vi "HFRR ADV v025 new software.vi"() -> ()   [LabVIEW 2025] (continued)
              n2926 = Greater?(x=w4117, y=1) -> (0:w4113:bool)
            }
            n2927 = local write "String 29"(w4094) -> ()
            n2928 = Search and Replace String(input string=w4094, search string=".duf", replace string=".dgf" ("replace string (\"\")")) -> (result string=→"String Indicator 4":string)  [unwired: 5 in, 3 out]
            n2929 = Match Pattern(string=w4109, regular expression=".dwm") -> (before substring=w4093:string)  [unwired: 1 in, 3 out]
            "String Indicator" <- w4093
            n2930 = Match Pattern(string=w4094, regular expression=".dwm" ("substring (\"\")")) -> (before substring=w4095:string)  [unwired: 1 in, 3 out]
            "String Indicator 3" <- w4095
            n2931 = local write "TITTLE 2"(w4093) -> ()
            n2932 = String To Path(string=w4095) -> (path=w4102:path)
            "path" <- w4102
            n2933 = call <vilib>:"Read Characters From File.vi"("file path (dialog if empty)"=w4102, "start of read offset (chars.:0)"=60 ("start of read offset (chars.: 0)")) -> ("character string"=→"String Indicator 2":string)  [unwired: 4 in, 3 out]
          }
        }
        n2934 = call <vilib>:"Query Available Printers.vi"() -> ("system configured printers"=w3794:string[])  [unwired: 9 in, 2 out]
        "System Configured Printers 2" <- w3794
        n2935 = local read "OK Button 16"() -> (w3791:bool)
        n2936 = case shown="True" "OK Button 16" {
          frame False {
          }
          frame True {
            n2937 = stacked-sequence {
              frame #0 {
                n2938 = local read "Numeric 16"() -> (w4119:i32)
                n2939 = local write "Numeric 10"(w4119) -> ()
              }
              frame #1 {
                n2940 = local read "String 29"() -> (w4122:string)
                n2941 = String To Path(string=w4122) -> (path=w4121:path)
                n2942 = Open/Create/Replace File "Open File"(file path (use dialog)=w4121) -> (refnum out=w4123:refnum<file>)  [unwired: 5 in, 2 out]
                n2943 = for {
                  N: 16 -> [_]
                  tunnel: w4123 -> [w4130]
                  i -> [w4126]
                  (unwired) TRUE ("line mode (F)")
                  n2944 = Read from Text File "Read File"(file (use dialog)=w4130) -> (text=w4124:string)  [unwired: 3 in, 3 out]
                  n2945 = Match Pattern(string=w4124, regular expression="(") -> (after substring=w4129:string)  [unwired: 1 in, 3 out]
                  n2946 = Match Pattern(string=w4129, regular expression=")") -> (before substring=w4125:string)  [unwired: 1 in, 3 out]
                  n2947 = case shown="1" w4126 {
                    tunnel: w4125 -> [w4131 w4132 _ _ w4133 w4134 w4135 w4137 w4139 w4141 w4143 w4145 w4147 w4149 _]
                    tunnel: w4124 -> [_ _ _ _ _ _ _ _ _ _ _ _ _ _ _]
                    frame 0 {
                      "TITTLE" <- w4131
                    }
                    frame 1 {
                      "Sample ID" <- w4132
                    }
                    frame 2 {
                    }
                    frame 3 {
                    }
                    frame 4 {
                      "Test Date" <- w4133
                    }
                    frame 5 {
                      "Tested by" <- w4134
                    }
                    frame 6 {
                      n2948 = Fract/Exp String To Number(string=w4135) -> (number=→"Humidity before test 2":dbl)  [unwired: 3 in, 1 out]
                    }
                    frame 7 {
                      n2949 = Fract/Exp String To Number(string=w4137) -> (number=→"Temperature before test 2":dbl)  [unwired: 3 in, 1 out]
                    }
                    frame 8 {
                      n2950 = Fract/Exp String To Number(string=w4139) -> (number=→"Humidity after test 2":dbl)  [unwired: 3 in, 1 out]
                    }
                    frame 9 {
                      n2951 = Fract/Exp String To Number(string=w4141) -> (number=→"Temperature after test 2":dbl)  [unwired: 3 in, 1 out]
                    }
                    frame 10 {
                      n2952 = Fract/Exp String To Number(string=w4143) -> (number=→"MWSD 2":dbl)  [unwired: 3 in, 1 out]
                    }
                    frame 11 {
                      n2953 = Fract/Exp String To Number(string=w4145) -> (number=→"AVP 2":dbl)  [unwired: 3 in, 1 out]
                    }
                    frame 12 {
                      n2954 = Fract/Exp String To Number(string=w4147) -> (number=→"HCF 2":dbl)  [unwired: 3 in, 1 out]
                    }
                    frame 13 {
                      n2955 = Fract/Exp String To Number(string=w4149) -> (number=→"WS1.4 2":dbl)  [unwired: 3 in, 1 out]
                    }
                    frame 14, Default {
                    }
                  }
                }
              }
              frame #2 {
              }
            }
            n2956 = local write "OK Button 16"(FALSE ("OK Button 13")) -> ()
          }
        }
        n2957 = Index Array(array=w3794, index="Select Printer 3") -> (element=w3796:string)
        "Selected Printer" <- w3796
        n2958 = case shown="True" w3791 {
          frame False {
          }
          frame True {
            n2959 = flat-sequence {
              frame #0 {
              }
              frame #1 {
                n2960 = Wait (ms)(milliseconds to wait=u32 100) -> ()  [unwired: 1 out]
              }
              frame #2 {
                n2961 = local write "OK Button 16"(FALSE ("Print 3")) -> ()
              }
            }
          }
        }
        n2962 = case shown="True" "Print" {
          tunnel: w3796 -> [_ w4088]
          frame False {
          }
          frame True {
            (unwired) i16 6 ("width (-)")
            (unwired) "TESTED BY : "
            (unwired) "TESTED DATE :"
            (unwired) "SAMPLE ID : "
            (unwired) "SAMPLE DESIGN : "
            w4046 = "\r"
            w4063 = "\r"
            # "add image"
            n2963 = local read "Sample ID"() -> (w4036:string)
            n2964 = local read "Tested by"() -> (w4039:string)
            n2965 = local read "String 34"() -> (w4026:string)
            n2966 = local read "String 45"() -> (w4006:string)
            n2967 = local read "String 35"() -> (w4021:string)
            n2968 = local read "String 37"() -> (w4019:string)
            n2969 = local read "String 32"() -> (w4041:string)
            n2970 = local read "String 36"() -> (w4016:string)
            n2971 = local read "String 31"() -> (w4040:string)
            n2972 = local read "Test Date"() -> (w4037:string)
            n2973 = local read "String 33"() -> (w4042:string)
            n2974 = local read "String 38"() -> (w4012:string)
            n2975 = local read "String 39"() -> (w4009:string)
            n2976 = local write "Print"(FALSE ("Print FF")) -> ()
            n2977 = local read "S 39"() -> (w4024:string)
            n2978 = local read "S 38"() -> (w4031:string)
            n2979 = local read "Temperature before test 2"() -> (w4062:dbl)
            n2980 = local read "Temperature after test 2"() -> (w4052:dbl)
            n2981 = local read "Humidity before test 2"() -> (w4077:dbl)
            n2982 = local read "Humidity after test 2"() -> (w4061:dbl)
            n2983 = local read "MWSD 2"() -> (w4066:dbl)
            n2984 = local read "WS1.4 2"() -> (w4044:dbl)
            n2985 = Concatenate Strings("2)" ("string"), w4026) -> (w4027:string)
            n2986 = Concatenate Strings("3)" ("string"), w4024) -> (w4025:string)
            n2987 = Concatenate Strings("1)" ("string"), w4031) -> (w4030:string)
            n2988 = Concatenate Strings("4)" ("string"), w4021) -> (w4022:string)
            n2989 = Concatenate Strings("5)" ("string"), w4019) -> (w4018:string)
            n2990 = Concatenate Strings("6)" ("string"), w4016) -> (w4015:string)
            n2991 = Concatenate Strings("7)" ("string"), w4012) -> (w4013:string)
            n2992 = Concatenate Strings("8)" ("string"), w4009) -> (w4010:string)
            n2993 = local read "HCF 2"() -> (w4048:dbl)
            n2994 = local read "AVP 2"() -> (w4065:dbl)
            n2995 = local read "s.NO"() -> (w4007:string)
            n2996 = call <vilib>:"New Report.vi"("report type"=enum16{"Standard Report", "HTML"}."Standard Report") -> ("report out"=w4086:refnum<class "NI_report.lvclass">, "error out"=w4085:errorcluster)  [unwired: 13 in]
            n2997 = local read "TITTLE"() -> (w4038:string)
            n2998 = Concatenate Strings(w4063, w4006, w4007, w4063, w4041, w4036, w4063, w4040, w4037, w4063, w4042, w4039, w4063) -> (w4056:string)
            "test by" <- w4056
            n2999 = Number To Fractional String(number=w4062, width (-)=i16 6, precision (6)=i16 2) -> (F-format string=w4051:string)  [unwired: 1 in]
            n3000 = Number To Fractional String(number=w4061, width (-)=i16 6, precision (6)=i16 2) -> (F-format string=w4064:string)  [unwired: 1 in]
            n3001 = Number To Fractional String(number=w4077, width (-)=i16 6, precision (6)=i16 2) -> (F-format string=w4082:string)  [unwired: 1 in]
            n3002 = Number To Fractional String(number=w4066, width (-)=i16 6, precision (6)=i16 2) -> (F-format string=w4068:string)  [unwired: 1 in]
            n3003 = Number To Fractional String(number=w4052, width (-)=i16 6, precision (6)=i16 2) -> (F-format string=w4053:string)  [unwired: 1 in]
            n3004 = Number To Fractional String(number=w4065, width (-)=i16 6, precision (6)=i16 2) -> (F-format string=w4067:string)  [unwired: 1 in]
            n3005 = Number To Fractional String(number=w4048, width (-)=i16 6, precision (6)=i16 2) -> (F-format string=w4047:string)  [unwired: 1 in]
            n3006 = Number To Fractional String(number=w4044, precision (6)=i16 2) -> (F-format string=w4043:string)  [unwired: 2 in]
            n3007 = call-dynamic "Set Report Header Text.vi"("report in"=w4086, "center header text"=w4038, "error in (no error)"=w4085) -> ("report out"=w4057:refnum<class "NI_report.lvclass">, "error out"=w4058:errorcluster)  [unwired: 11 in]
            n3008 = Concatenate Strings(w4046, w4030, w4082, w4046, w4027, w4051, w4046, w4025, w4064, w4046, w4022, w4053, w4046, w4018, w4068, w4046, w4015, w4067, w4046, w4013, w4047, w4046, w4010, w4043) -> (w4034:string)
            "export 2" <- w4034
            n3009 = call-poly <vilib>:"Append Report Text.vi"("report in"=w4057, "text"=w4056, "error in (no error)"=w4058) -> ("report out"=w4060:refnum<class "NI_report.lvclass">, "error out"=w4059:errorcluster)  [unwired: 9 in, 2 out]
            n3010 = local read "test by"() -> (w4033:string)
            n3011 = local read "TITTLE"() -> (w4035:string)
            n3012 = call-poly <vilib>:"Append Report Text.vi"("report in"=w4060, "error in (no error)"=w4059) -> ("report out"=w4081:refnum<class "NI_report.lvclass">, "error out"=w4079:errorcluster)  [unwired: 10 in, 2 out]
            n3013 = Concatenate Strings(w4035, w4034, w4033) -> (→"output":string)
            n3014 = call-poly <vilib>:"Append Report Text.vi"("report in"=w4081, "text"=w4034, "error in (no error)"=w4079) -> ("report out"=w4080:refnum<class "NI_report.lvclass">, "error out"=w4078:errorcluster)  [unwired: 9 in, 2 out]
            n3015 = call-dynamic "Print Report.vi"("report in"=w4080, "printer name (default)"=w4088, "error in (no error)"=w4078) -> ("report out"=w4090:refnum<class "NI_report.lvclass">, "error out"=w4091:errorcluster)  [unwired: 11 in]
            n3016 = call-dynamic "Dispose Report.vi"("report in"=w4090, "error in (no error)"=w4091) -> ()  [unwired: 13 in, 1 out]
          }
        }
        n3017 = case shown="True" "Print 2" {
          frame False {
          }
          frame True {
            n3018 = flat-sequence {
              frame #0 {
                n3019 = local read "s.NO"() -> (→"s.NO 2":string)
                n3020 = Wait (ms)(milliseconds to wait=u32 20) -> ()  [unwired: 1 out]
                n3021 = local read "Sample ID  3"() -> (→"Sample ID  6":string)
                n3022 = local read "Sample ID  4"() -> (→"Sample ID  7":string)
                n3023 = local read "Sample ID"() -> (→"Sample ID  2":string)
                n3024 = local read "Tested by"() -> (→"Tested by 2":string)
                n3025 = local read "Test Date"() -> (→"Test Date 2":string)
                n3026 = local read "Humidity after test 3"() -> (→"Humidity after test 4":dbl)
                n3027 = local read "Ref A Test Date :"() -> (→"TITTLE 4":string)
                n3028 = local read "Temperature before test 3"() -> (w3913:dbl)
                n3029 = local read "Temperature before test 3"() -> (→"Temperature after test 5":dbl)
                n3030 = local read "Temperature after test 3"() -> (→"Temperature after test 4":dbl)
                n3031 = local read "Humidity before test 3"() -> (→"Humidity before test 4":dbl)
                n3032 = local write "Temperature before test 3"(w3913) -> ()
                n3033 = local read "image data"() -> (w3904:T14)
                n3034 = String To Path(string="C:\\LAB-IQ\\im\\Temp_resized.jpg") -> (path=w3905:path)
                "path 2" <- w3905
                n3035 = call <vilib>:"Write JPEG File.vi"("image data"=w3904, "path to JPEG file"=w3905) -> ()  [unwired: 8 in, 2 out]
                "Ref A Test Date :" <- "Ref A Test Date :"
                "Ref B Test Date :" <- "Ref B Test Date :"
                "Ref B Scar Value :" <- "Ref B Scar Value :"
                "Ref A Scar Value :" <- "Ref A Scar Value :"
              }
              frame #1 {
                (unwired) HTML_Report_Image_Alignment."MIDDLE" ("alignment (default)")
                w3941 = u16 0 items=["portrait", "landscape"] ("orientation (portrait)")
                (unwired) HTML_Report_Image_Alignment."ABSMIDDLE" ("alignment (default)")
                (unwired) "TESTED BY : "
                (unwired) "TESTED DATE :"
                (unwired) "SAMPLE ID : "
                (unwired) "SAMPLE DESIGN : "
                w3974 = "\r"
                # "add image"
                n3036 = Wait (ms)(milliseconds to wait=u32 20) -> ()  [unwired: 1 out]
                n3037 = local read "Sample ID  2"() -> (w3967:string)
                n3038 = local read "Wear Scar X"() -> (w3939:dbl)
                "Length ( microns ) 2" <- w3939
                n3039 = local read "Wear Scar Y"() -> (w3938:dbl)
                "Wear Scar Y ( microns ) :" <- w3938
                n3040 = local read "Test Date 2"() -> (w3968:string)
                n3041 = local read "Tested by 2"() -> (w3969:string)
                n3042 = local read "String 46"() -> (w3965:string)
                n3043 = local read "String 48"() -> (w3971:string)
                n3044 = local read "String 47"() -> (w3970:string)
                n3045 = local read "String 49"() -> (w3972:string)
                n3046 = local read "String 10"() -> (w3925:string)
                n3047 = local read "s.NO 2"() -> (w3966:string)
                n3048 = Add(x=w3939, y=w3938) -> (x+y=w3937:dbl)
                n3049 = call <vilib>:"New Report.vi"("report type"=enum16{"Standard Report", "HTML"}."HTML") -> ("report out"=w3945:refnum<class "NI_report.lvclass">, "error out"=w3943:errorcluster)  [unwired: 13 in]
                n3050 = Concatenate Strings(w3974, w3965, w3966, w3974, w3971, w3967, w3974, w3970, w3968, w3974, w3972, w3969, w3974) -> (→"test by 2":string)
                n3051 = Concatenate Strings("C:\\LAB-IQ\\Data\\" ("string"), w3925, ".jpg" ("string")) -> ()  [unwired: 1 out]
                n3052 = Divide(x=w3937, y=2.0) -> (x/y=→"Mean Wear ( microns) :":dbl)
                n3053 = call-dynamic "Set Report Orientation.vi"("report in"=w3945, "orientation (portrait)"=w3941, "error in (no error)"=w3943) -> ("report out"=w3944:refnum<class "NI_report.lvclass">, "error out"=w3942:errorcluster)  [unwired: 11 in]
                n3054 = for {
                  N: 5 -> [_]
                  tunnel: w3944 -> [w3995]
                  tunnel: [w3994] -> w3923
                  tunnel: w3942 -> [w3993]
                  tunnel: [w3992] -> w3922
                  n3055 = call-dynamic "Set Report Tab Width.vi"("report in"=w3995, "error in (no error)"=w3993) -> ("report out"=w3994:refnum<class "NI_report.lvclass">, "error out"=w3992:errorcluster)  [unwired: 12 in]
                }
                n3056 = local read "TITTLE"() -> (w3940:string)
                n3057 = call-dynamic "Set Report Header Text.vi"("report in"=w3923, "center header text"=w3940, "error in (no error)"=w3922) -> ("report out"=w3961:refnum<class "NI_report.lvclass">, "error out"=w3960:errorcluster)  [unwired: 11 in]
                n3058 = for {
                  N: 1 -> [_]
                  tunnel: [w3999] -> w3947
                  tunnel: [w3998] -> w3946
                  tunnel: w3961 -> [w3997]
                  tunnel: w3960 -> [w3996]
                  n3059 = call-dynamic "New Report Line.vi"("report in"=w3997, "error in (no error)"=w3996) -> ("report out"=w3999:refnum<class "NI_report.lvclass">, "error out"=w3998:errorcluster)  [unwired: 12 in]
                }
                n3060 = for {
                  N: 2 -> [_]
                  tunnel: [w3991] -> w3953
                  tunnel: [w3990] -> w3952
                  tunnel: w3947 -> [w3989]
                  tunnel: w3946 -> [w3988]
                  n3061 = call-dynamic "New Report Line.vi"("report in"=w3989, "error in (no error)"=w3988) -> ("report out"=w3991:refnum<class "NI_report.lvclass">, "error out"=w3990:errorcluster)  [unwired: 12 in]
                }
                n3062 = for {
                  N: 25 -> [_]
                  tunnel: w3953 -> [w3987]
                  tunnel: w3952 -> [w3985]
                  tunnel: [w3986] -> w3956
                  tunnel: [w3984] -> w3955
                  n3063 = call-dynamic "Set Report Tab Width.vi"("report in"=w3987, "error in (no error)"=w3985) -> ("report out"=w3986:refnum<class "NI_report.lvclass">, "error out"=w3984:errorcluster)  [unwired: 12 in]
                }
                n3064 = control-ref of="Tab Control 9"() -> (w3951:refnum<vi>)
                n3065 = call-dynamic "Append Control Image to Report.vi"("report in"=w3956, "alignment (default)"=HTML_Report_Image_Alignment."ABSMIDDLE", "ctrl reference"=w3951, "error in (no error)"=w3955) -> ("report out"=w3950:refnum<class "NI_report.lvclass">, "error out"=w3949:errorcluster)  [unwired: 8 in, 2 out]
                n3066 = for {
                  N: 3 -> [_]
                  tunnel: [w3983] -> w3934
                  tunnel: [w3982] -> w3933
                  tunnel: w3950 -> [w3981]
                  tunnel: w3949 -> [w3980]
                  n3067 = call-dynamic "New Report Line.vi"("report in"=w3981, "error in (no error)"=w3980) -> ("report out"=w3983:refnum<class "NI_report.lvclass">, "error out"=w3982:errorcluster)  [unwired: 12 in]
                }
                n3068 = for {
                  N: 100 -> [_]
                  tunnel: w3934 -> [w3979]
                  tunnel: w3933 -> [w3977]
                  tunnel: [w3978] -> w3930
                  tunnel: [w3976] -> w3928
                  n3069 = call-dynamic "Set Report Tab Width.vi"("report in"=w3979, "error in (no error)"=w3977) -> ("report out"=w3978:refnum<class "NI_report.lvclass">, "error out"=w3976:errorcluster)  [unwired: 12 in]
                }
                n3070 = String To Path(string="C:\\LAB-IQ\\im\\Temp_resized.jpg") -> (path=w3920:path)
                n3071 = call-poly <vilib>:"Append Image to Report.vi"("report in"=w3930, "path or URL of image"=w3920, "error in (no error)"=w3928) -> ("report out"=w3929:refnum<class "NI_report.lvclass">, "error out"=w3927:errorcluster)  [unwired: 9 in, 2 out]
                n3072 = call-poly <vilib>:"Open HTML Report in Browser.vi"("report in"=w3929, "error in (no error)"=w3927) -> ("report out"=w3964:refnum<class "NI_report.lvclass">, "error out"=w3963:errorcluster)  [unwired: 11 in, 1 out]
                n3073 = call-dynamic "Dispose Report.vi"("report in"=w3964, "error in (no error)"=w3963) -> ()  [unwired: 13 in, 1 out]
              }
              frame #2 {
              }
              frame #3 {
                n3074 = disable-structure shown="Disabled" {
                  frame Disabled {
                    n3075 = local read "String 10"() -> (w4004:string)
                    n3076 = Concatenate Strings("C:\\LAB-IQ-NXT\\Data\\" ("string"), w4004, ".jpg" ("string")) -> (w4002:string)
                    n3077 = String To Path(string=w4002) -> (path=w4001:path)
                    n3078 = Delete(path (use dialog)=w4001) -> ()  [unwired: 4 in, 3 out]
                  }
                  frame Enabled {
                  }
                }
                n3079 = local write "Print 2"(FALSE ("Print")) -> ()
              }
            }
          }
        }
      }
    }
    n3080 = property on="SetTemp" class="DigNum (strict)"("Disabled"=w2100) -> ()  [unwired: 2 in, 2 out]
    n3081 = Multiply(x=w2090, y=w2092) -> (x*y=w2091:dbl)
    n3082 = local read "MWSD"() -> (w2089:dbl)
    n3083 = Add(x=w2091, y=w2089) -> (x+y=→"WS1.4":dbl)
    n3084 = Wait (ms)(milliseconds to wait=u32 50) -> ()  [unwired: 1 out]
    n3085 = Wait (ms)(milliseconds to wait=u32 50) -> ()  [unwired: 1 out]
    n3086 = local read "Quit"() -> (w2088:bool)
  }
  n3087 = VISA Close(VISA resource name=w41, error in (no error)=w40) -> ()  [unwired: 1 out]
  n3088 = while {
    tunnel: [w4164] -> w50
    shift-right: [w4157] -> _
    shift-left: 0.0 -> [w4160]
    shift-right: [w4156] -> _
    shift-left: 0.0 -> [w4159]
    shift-right: [w4155] -> _
    shift-left: 100.0 ("vc_cmd") -> [w4158]
    stop <- w4164 stop-if-true
    # "PID LOGIC"
    n3089 = local read "RUN"() -> (w4162:bool)
    n3090 = local read "Auto Start Temp"() -> (w4151:bool)
    n3091 = local read "Auto Start Test"() -> (w4161:bool)
    n3092 = local read "START TEMP"() -> (w4153:bool)
    n3093 = And(x=w4151, y=w4161) -> (x .and. y?=w4152:bool)
    n3094 = Or(x=w4162, y=w4152) -> (x .or. y?=w4163:bool)
    n3095 = And(x=w4163, y=w4153) -> (x .and. y?=w4154:bool)
    n3096 = Wait (ms)(milliseconds to wait="milliseconds to wait") -> ()  [unwired: 1 out]
    n3097 = case shown="True" w4154 {
      tunnel: [400.0 ("out_vc_cmd") w4184] -> w4155
      tunnel: [w4167 w4186] -> w4156
      tunnel: [w4167 w4185] -> w4157
      tunnel: w4160 -> [_ w4175]
      tunnel: w4159 -> [_ w4174]
      tunnel: w4158 -> [_ w4173]
      frame False {
        w4167 = 0.0 ("error_out")
      }
      frame True {
        n3098 = local read "Set Strk"() -> (w4170:dbl)
        n3099 = local read "LVDT STROKE"() -> (w4168:dbl)
        n3100 = Add(x=w4170, y="Add up Stroke") -> (x+y=w4171:dbl)
        n3101 = formula code="// Zero-Hardcode Explicit Positional-Form PID Engine\n// Inputs: target_stroke, measured_stroke, dt, prev_error, integral_accumulator_in, prev_vc_cmd\n//         kp, ki, kd, max_step_change, max_amplitude, min_amplitude, startup_cmd\n// Outputs: vc_cmd, error_out, out_error, integral_accumulator_out, out_vc_cmd\n\n// 1. Calculate Tracking Error\nfloat current_error = target_stroke - measured_stroke;\nerror_out = current_error;\n\n// 2. Compute Proportional Term\nfloat p_term = kp * current_error;\n\n// 3. Compute Derivative Term\nfloat d_term = 0.0;\nif (dt > 0.0) {\n    d_term = kd * ((current_error - prev_error) / dt);\n}\n\n// 4. Update and Accumulate Integral Term\nfloat current_integral = integral_accumulator_in + (current_error * dt);\nfloat i_term = ki * current_integral;\n\n// 5. Calculate Ideal Target Command\nfloat ideal_command = startup_cmd + p_term + i_term + d_term;\n\n// 6. Anti-Windup Protection (Back-calculation method)\nif (ideal_command > max_amplitude) {\n    float excess = ideal_command - max_amplitude;\n    if (ki > 0.0) {\n        current_integral -= excess / ki;\n    }\n    ideal_command = max_amplitude;\n} else if (ideal_command < min_amplitude) {\n    float excess = ideal_command - min_amplitude;\n    if (ki > 0.0) {\n        current_integral -= excess / ki;\n    }\n    ideal_command = min_amplitude;\n}\n\n// 7. Apply Loop Rate Limiting (Protects voice coil from large voltage steps)\nfloat raw_adjustment = ideal_command - prev_vc_cmd;\n\nif (raw_adjustment > max_step_change) {\n    raw_adjustment = max_step_change;\n} else if (raw_adjustment < -max_step_change) {\n    raw_adjustment = -max_step_change;\n}\n\nfloat next_vc_cmd = prev_vc_cmd + raw_adjustment;\n\n// Final Output Safety Safeguard Clamping\nif (next_vc_cmd > max_amplitude) {\n    next_vc_cmd = max_amplitude;\n} else if (next_vc_cmd < min_amplitude) {\n    next_vc_cmd = min_amplitude;\n}\n\n// 8. Map to Shift Registers for memory persistence\nvc_cmd = next_vc_cmd;\nout_error = current_error;                     \nintegral_accumulator_out = current_integral;  \nout_vc_cmd = next_vc_cmd;"("target_stroke"=w4171, "measured_stroke"=w4168, "dt"="dt", "integral_accumulator_in"=w4174, "prev_error"=w4175, "prev_vc_cmd"=w4173, "kp"="kp", "ki"="ki", "kd"="kd", "max_step_change"="max_step_change", "max_amplitude"="max_amplitude", "min_amplitude"="min_amplitude", "startup_cmd"="startup_cmd") -> ("vc_cmd"=w4190:dbl, "out_error"=w4185:dbl, "integral_accumulator_out"=w4186:dbl, "out_vc_cmd"=w4184:dbl)  [unwired: 1 out]
        "output Vpp" <- w4190
        n3102 = Number To Fractional String(number=w4190, precision (6)=i16 1) -> (F-format string=w4188:string)  [unwired: 2 in]
        n3103 = Concatenate Strings("DAC;" ("string"), w4188) -> (w4172:string)
        n3104 = local write "Due Write"(w4172) -> ()
        "prev_error" <- w4175
        "integral_accumulator_in" <- w4174
        "prev_vc_cmd" <- w4173
      }
    }
    n3105 = local read "Quit"() -> (w4164:bool)
  }
  n3106 = Or(x=w46, y=w45) -> (x .or. y?=w47:bool)
  n3107 = Or(x=w43, y=w47) -> (x .or. y?=w52:bool)
  n3108 = control-ref of="new picture"() -> ()  [unwired: 1 out]
  n3109 = Or(x=w55, y=w52) -> (x .or. y?=w49:bool)
  n3110 = Or(x=w49, y=w50) -> (x .or. y?=w44:bool)
  n3111 = while {
    tunnel: [w4191] -> w54
    i -> [w4198]
    stop <- w4191 stop-if-true
    n3112 = local read "Quit"() -> (w4191:bool)
    n3113 = Equal To 0?(x=w4198) -> (x = 0?=w4196:bool)
    n3114 = call "Elapsed Time3"("Time Target (s)"=45.0, "Auto Reset"=TRUE) -> ("Time has Elapsed"=w4195:bool)  [unwired: 10 in, 7 out]
    n3115 = Wait (ms)(milliseconds to wait=u32 50) -> ()  [unwired: 1 out]
    n3116 = Or(x=w4195, y=w4196) -> (x .or. y?=w4197:bool)
    n3117 = case shown="True" w4197 {
      frame False {
      }
      frame True {
        n3118 = call <vilib>:"System Exec.vi"("run minimized? (F)"=TRUE, "error in (no error)"="error in (no error)", "command line"="powercfg.exe -change -monitor-timeout-ac 0") -> ("error out"=w4209:errorcluster)  [unwired: 5 in, 3 out]
        n3119 = call <vilib>:"System Exec.vi"("run minimized? (F)"=TRUE, "error in (no error)"=w4209, "command line"="powercfg.exe -change -disk-timeout-ac 0") -> ("error out"=w4208:errorcluster)  [unwired: 5 in, 3 out]
        n3120 = call <vilib>:"System Exec.vi"("run minimized? (F)"=TRUE, "error in (no error)"=w4208, "command line"="powercfg.exe -change -standby-timeout-ac 0") -> ("error out"=w4207:errorcluster)  [unwired: 5 in, 3 out]
        n3121 = call <vilib>:"System Exec.vi"("run minimized? (F)"=TRUE, "error in (no error)"=w4207, "command line"="powercfg.exe -change -hibernate-timeout-ac 0") -> ("error out"=w4206:errorcluster)  [unwired: 5 in, 3 out]
        n3122 = call <vilib>:"Simple Error Handler.vi"("error in (no error)"=w4206) -> ("error out"=w4212:errorcluster)  [unwired: 4 in, 4 out]
        n3123 = call <vilib>:"Clear Errors.vi"("error in (no error)"=w4212) -> ("error out"=→"error out":errorcluster)  [unwired: 5 in, 1 out]
      }
    }
  }
  n3124 = Compound Arithmetic op=OR(w57, w44, w54) -> (w56:bool)
  n3125 = flat-sequence {
    tunnel: w56 -> [_]
    tunnel: [w4214] -> w25
    tunnel: w25 -> [_]
    frame #0 {
      n3126 = call "CLOSE CONNECTION.vi"() -> ("error out"=w4214:errorcluster)  [unwired: 11 in]
    }
    frame #1 {
      n3127 = Quit LabVIEW(quit? (T)=TRUE) -> ()
      n3128 = local write "Quit"(FALSE ("EXIT")) -> ()
    }
  }
  n3129 = property on="Heater Button" class="Bool (strict)"("Visible"=TRUE) -> ()  [unwired: 2 in, 2 out]
  n3130 = disable-structure shown="Disabled" {
    disable-tunnel: _ -> [w4220 _]
    disable-tunnel: _ -> [w4217 _]
    disable-tunnel: _ -> [w4218 _]
    frame Disabled {
      n3131 = disable-structure shown="Disabled" {
        disable-tunnel: [w4227 _] -> w4219
        frame Disabled {
          n3132 = while {
            shift-right: [w4269] -> w4225
            shift-left: errorcluster {"status"=TRUE, "code"=0, "source"="Init"} ("error out") -> [w4234]
            shift-right: [w4268] -> w4224
            shift-left: _ -> [w4235]
            shift-right: [w4267] -> _
            shift-left: "" -> [w4266]
            tunnel: [w4228] -> w4227
            shift-right: ["Set Rh"] -> _
            shift-left: 0.0 ("Set Rh") -> [w4260]
            tunnel: [w4237] -> _
            i -> [w4237]
            stop <- w4228 stop-if-true
            n3133 = flat-sequence {
              tunnel: w4234 -> [w4272]
              tunnel: [w4272] -> w4233
              frame #0 {
                n3134 = Wait (ms)(milliseconds to wait=u32 200) -> ()  [unwired: 1 out]
              }
            }
            n3135 = local read "Com Port 3"() -> (w4236:refnum<visa-resource-name>)
            n3136 = local read "Humidity Str Rec"() -> (w4238:string)
            n3137 = Not Equal?(x="Set Rh", y=w4260) -> (x != y?=w4265:bool)
            n3138 = Number To Decimal String(number="Set Rh") -> (decimal integer string=w4263:string)  [unwired: 1 in]
            n3139 = Not Equal?(x=w4236, y=w4235) -> (x != y?=w4231:bool)
            n3140 = Concatenate Strings("#setPoint00" ("string"), w4263) -> (w4264:string)
            n3141 = case shown="False" w4265 {
              tunnel: w4264 -> [_ w4284]
              frame False {
                n3142 = local read "Humidity"() -> (w4281:bool)
                n3143 = case shown="True" w4281 {
                  frame False {
                    n3144 = local write "Humidity Str Send"("stop" ("Humidity Str Send")) -> ()
                  }
                  frame True {
                    n3145 = local write "Humidity Str Send"("start" ("Humidity Str Send")) -> ()
                  }
                }
              }
              frame True {
                n3146 = local write "Humidity Str Send"(w4284) -> ()
              }
            }
            n3147 = Or(x=w4231) -> (y=w4229:bool, x .or. y?=w4230:bool)
            n3148 = String Subset(string=w4238, offset (0)=7) -> (substring=w4253:string)  [unwired: 1 in]
            n3149 = Match Pattern(string=w4238, regular expression="?") -> (offset past match=w4256:i32)  [unwired: 1 in, 3 out]
            n3150 = Match Pattern(string=w4238, regular expression="v") -> (offset past match=w4259:i32)  [unwired: 1 in, 3 out]
            n3151 = case shown="True" w4230 {
              tunnel: w4233 -> [w4270 _]
              tunnel: [w4270 errorcluster {"status"=TRUE, "code"=0, "source"="Init"} ("error out")] -> w4232
              frame False {
              }
              frame True {
              }
            }
            n3152 = Equal?(x=w4256, y=-1) -> (x = y?=w4240:bool)
            n3153 = Match Pattern(string=w4253, regular expression="g") -> (after substring=w4254:string, offset past match=w4245:i32)  [unwired: 1 in, 2 out]
            n3154 = Match Pattern(string=w4253, regular expression="y") -> (after substring=w4252:string, offset past match=w4246:i32)  [unwired: 1 in, 2 out]
            n3155 = Greater?(x=w4246, y=w4245) -> (0:w4251:bool)
            n3156 = Greater Or Equal To 0?(x=w4246) -> (x >= 0?=w4243:bool)
            n3157 = Greater Or Equal To 0?(x=w4245) -> (x >= 0?=w4244:bool)
            n3158 = Or(x=w4243, y=w4244) -> (x .or. y?=w4242:bool)
            n3159 = Greater Or Equal To 0?(x=w4259) -> (x >= 0?=w4241:bool)
            n3160 = Select(t=w4252, s=w4251, f=w4254) -> (s? t:f=w4247:string)
            n3161 = case shown="Error" w4232 {
              selector: w4232 -> [w4297 w4343]
              tunnel: [w4295 w4336] -> w4269
              tunnel: w4235 -> [w4298 w4342]
              tunnel: [w4296 w4345] -> w4268
              tunnel: w4266 -> [w4285 w4344]
              tunnel: [w4292 w4344] -> w4267
              frame No Error {
                n3162 = call "Elapsed Time7"() -> ("Time has Elapsed"=w4291:bool)  [unwired: 12 in, 7 out]
                n3163 = Not Equal?(x="Humidity Str Send", y=w4285) -> (x != y?=w4287:bool)
                n3164 = Or(x=w4287, y=w4291) -> (x .or. y?=w4290:bool)
                n3165 = Select(t="Humidity Str Send", s=w4287, f="vals" ("regular expression")) -> (s? t:f=w4286:string)
                n3166 = Or(x=w4290, y="Send") -> (x .or. y?=w4294:bool)
                n3167 = case shown="True" w4294 {
                  tunnel: [w4301 w4306] -> w4295
                  tunnel: w4298 -> [w4300 w4314]
                  tunnel: w4297 -> [w4301 w4313]
                  tunnel: [w4300 w4307] -> w4296
                  tunnel: w4286 -> [_ w4312]
                  tunnel: [w4299 w4303] -> w4292
                  tunnel: "Humidity Str Send" -> [_ w4304]
                  tunnel: w4287 -> [_ w4305]
                  tunnel: w4285 -> [w4299 w4302]
                  frame False {
                  }
                  frame True {
                    n3168 = flat-sequence {
                      tunnel: w4314 -> [w4322]
                      tunnel: w4313 -> [w4321]
                      tunnel: w4312 -> [w4318]
                      tunnel: [w4320] -> w4311
                      tunnel: [w4319] -> w4310
                      tunnel: w4311 -> [w4325]
                      tunnel: w4310 -> [w4324]
                      tunnel: [w4325] -> w4309
                      tunnel: [w4324] -> w4308
                      tunnel: w4309 -> [w4332]
                      tunnel: w4308 -> [w4331]
                      tunnel: [w4330] -> w4307
                      tunnel: [w4329] -> w4306
                      frame #0 {
                        n3169 = local write "Ser Led"(TRUE ("Boolean 4")) -> ()
                        n3170 = Concatenate Strings(w4318, "\r") -> (w4317:string)
                        n3171 = VISA Write(VISA resource name=w4322, write buffer=w4317, error in (no error)=w4321) -> (VISA resource name out=w4320:refnum<visa-resource-name>, error out=w4319:errorcluster)  [unwired: 1 out]
                      }
                      frame #1 {
                        n3172 = Wait (ms)(milliseconds to wait="wait") -> ()  [unwired: 1 out]
                      }
                      frame #2 {
                        w4327 = FALSE ("Send")
                        n3173 = property class="Instr"(reference=w4332, error in=w4331) -> (reference out=w4333:refnum<visa-resource-name>, error out=w4334:errorcluster, "Serial Settings:Number of Bytes at Serial Port"=w4326:u32)
                        n3174 = local write "Send"(w4327) -> ()
                        n3175 = local write "Ser Led"(w4327) -> ()
                        n3176 = VISA Read(VISA resource name=w4333, byte count=w4326, error in (no error)=w4334) -> (VISA resource name out=w4330:refnum<visa-resource-name>, read buffer=→"Humidity Str Rec":string, error out=w4329:errorcluster)  [unwired: 1 out]
                      }
                    }
                    n3177 = Select(t=w4304, s=w4305, f=w4302) -> (s? t:f=w4303:string)
                  }
                }
              }
              frame Error {
                w4350 = u16 0 items=["None"=0, "XON/XOFF"=1, "RTS/CTS"=2, "DTR/DSR"=4] ("flow control")
                w4346 = u16 0 items=["None", "Odd", "Even", "Mark", "Space"] ("parity")
                w4349 = u16 10 items=["1.0"=10, "1.5"=15, "2.0"=20] ("stop bits")
                n3178 = VISA Close(VISA resource name=w4342, error in (no error)=w4343) -> (error out=w4341:errorcluster)
                n3179 = local write "humid"("" ("humid")) -> ()
                n3180 = local write "Humidity Str Rec"("" ("Humidity Str Rec")) -> ()
                n3181 = call <vilib>:"Clear Errors.vi"("error in (no error)"=w4341) -> ("error out"=w4340:errorcluster)  [unwired: 5 in, 1 out]
                n3182 = local read "Com Port 3"() -> (w4339:refnum<visa-resource-name>)
                n3183 = call-poly "VISA Configure Serial Port"("VISA resource name"=w4339, "timeout (10sec)"=u32 1000, "termination char\n(0xA = '\\n' = LF)"=u8 10 ("termination char\n(0xA = '\\n' = LF)"), "Enable Termination\nChar (T)"=FALSE ("Enable Termination Char (T)"), "data bits (8)"=u16 8 ("data bits"), "parity (0:none)"=w4346, "error in (no error)"=w4340, "stop bits (10: 1 bit)"=w4349, "flow control (0:none)"=w4350) -> ("VISA resource name out"=w4345:refnum<visa-resource-name>, "baud rate (9600)"=w4337:u32, "error out"=w4336:errorcluster)  [unwired: 4 in]
              }
            }
            n3184 = Compound Arithmetic op=AND(w4241, w4240, w4242) -> (w4239:bool)
            n3185 = case shown="True" w4239 {
              tunnel: w4238 -> [_ _]
              tunnel: w4247 -> [_ w4277]
              frame False {
              }
              frame True {
                w4275 = " " ("regular expression")
                n3186 = Match Pattern(string=w4277, regular expression=" ") -> (after substring=w4279:string)  [unwired: 1 in, 3 out]
                n3187 = Match Pattern(string=w4279, regular expression=w4275) -> (before substring=→"humid":string, after substring=w4276:string)  [unwired: 1 in, 2 out]
                n3188 = Match Pattern(string=w4276, regular expression=w4275) -> (before substring=→"temp_@Rh sensor":string)  [unwired: 1 in, 3 out]
              }
            }
            n3189 = local read "Quit"() -> (w4228:bool)
          }
          n3190 = VISA Close(VISA resource name=w4224, error in (no error)=w4225) -> (error out=w4221:errorcluster)
          n3191 = call <vilib>:"Clear Errors.vi"("error in (no error)"=w4221) -> ()  [unwired: 5 in, 2 out]
        }
        frame Enabled {
        }
      }
    }
    frame Enabled {
    }
  }
  n3192 = while {
    tunnel: [w4357] -> _
    i -> [w4357]
    stop <- w4353 stop-if-true
    # "Langauage selection"
    n3193 = Equal?(x="Lan flag", y=22.0) -> ()  [unwired: 1 out]
    n3194 = disable-structure shown="Disabled" {
      frame Disabled {
        n3195 = stacked-sequence {
          frame #0 {
            n3196 = case shown="\"Russian\"" "Language Selection" {
              tunnel: [0 1] -> w4359
              frame "English", Default {
              }
              frame "Russian" {
              }
            }
            n3197 = for {
              N: 130 -> [_]
              tunnel: "Table" -> [w4368]
              tunnel: w4359 -> [w4367]
              i -> [w4366]
              n3198 = Index Array(array=w4368, index (row)=w4366, index (col)=w4367) -> (element=w4365:string)
              n3199 = case shown="123" w4366 {
                tunnel: w4365 -> [w4369 w4370 _ w4371 w4372 w4373 w4374 w4375 w4376 w4377 w4378 w4379 w4380 w4381 w4382 w4383 w4384 w4385 w4386 w4387 w4388 w4389 w4390 w4391 w4392 w4393 w4394 w4395 w4396 _ _ w4397 w4398 w4399 w4400 w4401 w4402 w4411 w4418 w4425 w4432 w4436 w4439 w4442 w4444 w4446 w4447 w4448 w4449 w4450 w4451 w4452 w4453 w4454 w4455 w4456 w4457 w4458 w4459 w4460 w4461 w4462 w4463 w4464 w4465 w4466 w4467 w4468 w4469 w4470 w4471 w4472 w4473 w4474 w4475 w4476 w4477 w4478 w4479 w4480 w4481 w4482 w4483 w4484 w4485 w4486 w4487 w4488 w4489 w4490 w4491 w4492 w4493 w4494 w4495 w4496 w4497 w4498 w4499 w4500 w4501 w4502 w4503 w4504 w4505 _ w4506 w4507 w4508 w4509 w4510 w4511 w4512 w4513 w4514 w4515 w4516 w4517 w4518 _ w4519 w4520 w4521 w4522 w4523 w4524 _]
                frame 0 {
                  n3200 = local write "S"(w4369) -> ()
                }
                frame 1 {
                  n3201 = local write "S 2"(w4370) -> ()
                }
                frame 2 {
                }
                frame 3 {
                  n3202 = local write "S 4"(w4371) -> ()
                }
                frame 4 {
                  n3203 = property on="FILE" class="Str"("Caption.Text"=w4372) -> ()  [unwired: 2 in, 2 out]
                }
                frame 5 {
                  n3204 = property on="Fuel Discription :" class="Str"("Caption.Text"=w4373) -> ()  [unwired: 2 in, 2 out]
                }
                frame 6 {
                  n3205 = property on="Remarks :" class="Str"("Caption.Text"=w4374) -> ()  [unwired: 2 in, 2 out]
                }
                frame 7 {
                  n3206 = property on="Save & Continue" class="Bool (strict)"("Boolean Text.Text"=w4375) -> ()  [unwired: 2 in, 2 out]
                }
                frame 8 {
                }
                frame 9 {
                  n3207 = property on="Set Hz" class="DigNum (strict)"("Caption.Text"=w4377) -> ()  [unwired: 2 in, 2 out]
                }
                frame 10 {
                }
                frame 11 {
                  n3208 = property on="NORMAL LOAD" class="DigNum (strict)"("Caption.Text"=w4379) -> ()  [unwired: 2 in, 2 out]
                }
                frame 12 {
                }
                frame 13 {
                  n3209 = property on="Set Temp" class="DigNum (strict)"("Caption.Text"=w4381) -> ()  [unwired: 2 in, 2 out]
                }
                frame 14 {
                  n3210 = local write "S 15"(w4382) -> ()
                }
                frame 15 {
                  n3211 = property on="Set Rh" class="DigNum (strict)"("Caption.Text"=w4383) -> ()  [unwired: 2 in, 2 out]
                }
                frame 16 {
                }
                frame 17 {
                  n3212 = local write "S 18"(w4385) -> ()
                }
                frame 18 {
                  "String 17" <- w4386
                }
                frame 19 {
                  n3213 = property on="test time" class="DigNum (strict)"("Caption.Text"=w4387) -> ()  [unwired: 2 in, 2 out]
                }
                frame 20 {
                  "String 18" <- w4388
                  "String 22" <- w4388
                }
                frame 21 {
                  n3214 = property on="Elapsed time" class="DigNum (strict)"("Caption.Text"=w4389) -> ()  [unwired: 2 in, 2 out]
                }
                frame 22 {
                  n3215 = property on="Samplingtime 2" class="DigNum (strict)"("Caption.Text"=w4390) -> ()  [unwired: 2 in, 2 out]
                }
                frame 23 {
                  "String 21" <- w4391
                }
                frame 24 {
                  n3216 = property on="Countdown" class="DigNum (strict)"("Caption.Text"=w4392) -> ()  [unwired: 2 in, 2 out]
                }
                frame 25 {
                  n3217 = property on="Countdown 2" class="DigNum (strict)"("Caption.Text"=w4393) -> ()  [unwired: 2 in, 2 out]
                }
                frame 26 {
                  n3218 = property on="Engage" class="Bool (strict)"("Boolean Text.Text"=w4394) -> ()  [unwired: 2 in, 2 out]
                }
                frame 27 {
                  n3219 = property on="Boolean  4" class="Bool (strict)"("Boolean Text.Text"=w4395) -> ()  [unwired: 2 in, 2 out]
                }
                frame 28 {
                  n3220 = property on="Test \nStatus" class="Bool (strict)"("Boolean Text.Text"=w4396) -> ()  [unwired: 2 in, 2 out]
                }
                frame 29 {
                }
                frame 30 {
                }
                frame 31 {
                }
                frame 32 {
                  n3221 = property on="RSTCOF" class="Bool"("Boolean Text.Text"=w4398) -> ()  [unwired: 2 in, 2 out]
                  n3222 = property on="RST FF" class="Bool"("Boolean Text.Text"=w4398) -> ()  [unwired: 2 in, 2 out]
                  n3223 = property on="RST TEMP" class="Bool"("Boolean Text.Text"=w4398) -> ()  [unwired: 2 in, 2 out]
                  n3224 = property on="RSTV1 3" class="Bool"("Boolean Text.Text"=w4398) -> ()  [unwired: 2 in, 2 out]
                  n3225 = property on="rstv2" class="Bool"("Boolean Text.Text"=w4398) -> ()  [unwired: 2 in, 2 out]
                  n3226 = property on="RSTV1 2" class="Bool"("Boolean Text.Text"=w4398) -> ()  [unwired: 2 in, 2 out]
                  n3227 = property on="RST CP" class="Bool"("Boolean Text.Text"=w4398) -> ()  [unwired: 2 in, 2 out]
                }
                frame 33 {
                  "S 61" <- w4399
                }
                frame 34 {
                  "String 23" <- w4400
                }
                frame 35 {
                  n3228 = property on="Rh Before" class="DigNum (strict)"("Caption.Text"=w4401) -> ()  [unwired: 2 in, 2 out]
                }
                frame 36 {
                  n3229 = Match Pattern(string=w4402, regular expression=",") -> (before substring=→"bs":string, after substring=→"as":string)  [unwired: 1 in, 2 out]
                  n3230 = property on="Rh After" class="DigNum (strict)"("Caption.Text"=w4402) -> ()  [unwired: 2 in, 2 out]
                }
                frame 37 {
                  n3231 = Match Pattern(string=w4411, regular expression=",") -> (before substring=w4410:string, after substring=w4409:string)  [unwired: 1 in, 2 out]
                  "bs" <- w4410
                  "as" <- w4409
                  n3232 = Concatenate Strings(w4410, w4409) -> (w4406:string)
                  n3233 = property on="Humidity before test 2" class="DigNum (strict)"("Caption.Text"=w4406) -> ()  [unwired: 2 in, 2 out]
                  n3234 = property on="Humidity before test" class="DigNum (strict)"("Caption.Text"=w4406) -> ()  [unwired: 2 in, 2 out]
                  n3235 = Concatenate Strings(w4406, "=" ("string")) -> (w4407:string)
                  n3236 = local write "S 38"(w4407) -> ()
                }
                frame 38 {
                  n3237 = Match Pattern(string=w4418, regular expression=",") -> (before substring=w4417:string, after substring=w4416:string)  [unwired: 1 in, 2 out]
                  "bs" <- w4417
                  "as" <- w4416
                  n3238 = Concatenate Strings(w4417, w4416) -> (w4413:string)
                  n3239 = property on="Humidity after test 2" class="DigNum (strict)"("Caption.Text"=w4413) -> ()  [unwired: 2 in, 2 out]
                  n3240 = Concatenate Strings(w4413, "=" ("string")) -> (w4415:string)
                  n3241 = property on="Humidity after test" class="DigNum (strict)"("Caption.Text"=w4413) -> ()  [unwired: 2 in, 2 out]
                  n3242 = local write "S 39"(w4415) -> ()
                }
                frame 39 {
                  n3243 = Match Pattern(string=w4425, regular expression=",") -> (before substring=w4424:string, after substring=w4423:string)  [unwired: 1 in, 2 out]
                  "bs" <- w4424
                  "as" <- w4423
                  n3244 = Concatenate Strings(w4424, w4423) -> (w4420:string)
                  n3245 = property on="Temperature before test 2" class="DigNum (strict)"("Caption.Text"=w4420) -> ()  [unwired: 2 in, 2 out]
                  n3246 = property on="Temperature before test" class="DigNum (strict)"("Caption.Text"=w4420) -> ()  [unwired: 2 in, 2 out]
                  n3247 = Concatenate Strings(w4420, "=" ("string")) -> (→"String 34":string)
                }
                frame 40 {
                  n3248 = Match Pattern(string=w4432, regular expression=",") -> (before substring=w4431:string, after substring=w4430:string)  [unwired: 1 in, 2 out]
                  "bs" <- w4431
                  "as" <- w4430
                  n3249 = Concatenate Strings(w4431, w4430) -> (w4427:string)
                  n3250 = property on="Temperature after test 2" class="DigNum (strict)"("Caption.Text"=w4427) -> ()  [unwired: 2 in, 2 out]
                  n3251 = Concatenate Strings(w4427, "=" ("string")) -> (→"String 35":string)
                  n3252 = property on="Temperature after test" class="DigNum (strict)"("Caption.Text"=w4427) -> ()  [unwired: 2 in, 2 out]
                }
                frame 41 {
                  n3253 = property on="AVP" class="DigNum (strict)"("Caption.Text"=w4436) -> ()  [unwired: 2 in, 2 out]
                  n3254 = property on="AVP 2" class="DigNum (strict)"("Caption.Text"=w4436) -> ()  [unwired: 2 in, 2 out]
                  n3255 = Concatenate Strings(w4436, "=" ("string")) -> (→"String 36":string)
                }
                frame 42 {
                  n3256 = property on="MWSD" class="DigNum (strict)"("Caption.Text"=w4439) -> ()  [unwired: 2 in, 2 out]
                  n3257 = property on="MWSD 2" class="DigNum (strict)"("Caption.Text"=w4439) -> ()  [unwired: 2 in, 2 out]
                  n3258 = Concatenate Strings(w4439, "=" ("string")) -> (→"String 37":string)
                }
                frame 43 {
                  n3259 = property on="HCF 2" class="DigNum (strict)"("Caption.Text"=w4442) -> ()  [unwired: 2 in, 2 out]
                  n3260 = property on="HCF" class="DigNum (strict)"("Caption.Text"=w4442) -> ()  [unwired: 2 in, 2 out]
                  n3261 = Concatenate Strings(w4442, "=" ("string")) -> (→"String 38":string)
                }
                frame 44 {
                  n3262 = Concatenate Strings(w4444, "=" ("string")) -> (→"String 39":string)
                  n3263 = property on="WS1.4 2" class="DigNum (strict)"("Caption.Text"=w4444) -> ()  [unwired: 2 in, 2 out]
                  n3264 = property on="WS1.4" class="DigNum (strict)"("Caption.Text"=w4444) -> ()  [unwired: 2 in, 2 out]
                }
                frame 45 {
                  n3265 = property on="Save Results" class="Bool (strict)"("Boolean Text.Text"=w4446) -> ()  [unwired: 2 in, 2 out]
                }
                frame 46 {
                  n3266 = local write "S 47"(w4447) -> ()
                }
                frame 47 {
                  n3267 = local write "S 48"(w4448) -> ()
                }
                frame 48 {
                  n3268 = local write "S 49"(w4449) -> ()
                }
                frame 49 {
                  n3269 = local write "S 50"(w4450) -> ()
                }
                frame 50 {
                  n3270 = local write "S 51"(w4451) -> ()
                }
                frame 51 {
                  n3271 = local write "S 52"(w4452) -> ()
                }
                frame 52 {
                  n3272 = local write "S 53"(w4453) -> ()
                }
                frame 53 {
                  n3273 = local write "S 54"(w4454) -> ()
                }
                frame 54 {
                  n3274 = local write "S 55"(w4455) -> ()
                }
                frame 55 {
                  n3275 = local write "S 56"(w4456) -> ()
                }
                frame 56 {
                  n3276 = local write "S 57"(w4457) -> ()
                }
                frame 57 {
                  n3277 = local write "S 58"(w4458) -> ()
                }
                frame 58 {
                  n3278 = local write "S 59"(w4459) -> ()
                }
                frame 59 {
                  n3279 = local write "S 60"(w4460) -> ()
                }
                frame 60 {
                  n3280 = local write "S 62"(w4461) -> ()
                }
                frame 61 {
                  n3281 = local write "S 63"(w4462) -> ()
                }
                frame 62 {
                  n3282 = local write "S 64"(w4463) -> ()
                }
                frame 63 {
                  n3283 = local write "S 65"(w4464) -> ()
                }
                frame 64 {
                  n3284 = local write "S 66"(w4465) -> ()
                }
                frame 65 {
                  n3285 = local write "S 67"(w4466) -> ()
                }
                frame 66 {
                  n3286 = local write "S 68"(w4467) -> ()
                }
                frame 67 {
                  n3287 = local write "S 69"(w4468) -> ()
                }
                frame 68 {
                  n3288 = local write "S 70"(w4469) -> ()
                }
                frame 69 {
                  n3289 = local write "S 71"(w4470) -> ()
                }
                frame 70 {
                  n3290 = local write "S 72"(w4471) -> ()
                }
                frame 71 {
                  n3291 = local write "S 73"(w4472) -> ()
                }
                frame 72 {
                  n3292 = local write "S 74"(w4473) -> ()
                }
                frame 73 {
                  n3293 = local write "S 75"(w4474) -> ()
                }
                frame 74 {
                  n3294 = local write "S 76"(w4475) -> ()
                }
                frame 75 {
                  n3295 = local write "S 77"(w4476) -> ()
                }
                frame 76 {
                  n3296 = local write "S 78"(w4477) -> ()
                }
                frame 77 {
                  n3297 = local write "S 79"(w4478) -> ()
                }
                frame 79 {
                  n3298 = property on="Sample Temperature ( °C )" class="XYGraph (strict)"("Y Scale.Name Label.Text"=w4479) -> ()  [unwired: 2 in, 2 out]
                }
                frame 80 {
                  n3299 = local write "S 81"(w4480) -> ()
                  n3300 = property on="Humidity ( %RH )" class="XYGraph (strict)"("Y Scale.Name Label.Text"=w4480) -> ()  [unwired: 2 in, 2 out]
                }
                frame 78 {
                  n3301 = property on="Air Temperature  ( °C )" class="XYGraph (strict)"("X Scale.Name Label.Text"=w4481) -> ()  [unwired: 2 in, 2 out]
                  n3302 = property on="Humidity ( %RH )" class="XYGraph (strict)"("X Scale.Name Label.Text"=w4481) -> ()  [unwired: 2 in, 2 out]
                  n3303 = property on="Sample Temperature ( °C )" class="XYGraph (strict)"("X Scale.Name Label.Text"=w4481) -> ()  [unwired: 2 in, 2 out]
                  n3304 = property on="Coefficient Of Friction" class="XYGraph (strict)"("X Scale.Name Label.Text"=w4481) -> ()  [unwired: 2 in, 2 out]
                }
                frame 81 {
                  n3305 = property on="Air Temperature  ( °C )" class="XYGraph (strict)"("Y Scale.Name Label.Text"=w4482) -> ()  [unwired: 2 in, 2 out]
                }
                frame 82 {
                  n3306 = local write "S 84"(w4483) -> ()
                }
                frame 83 {
                  n3307 = local write "S 85"(w4484) -> ()
                }
                frame 84 {
                  n3308 = local write "S 86"(w4485) -> ()
                }
                frame 85 {
                  n3309 = local write "S 87"(w4486) -> ()
                }
                frame 86 {
                  n3310 = local write "S 88"(w4487) -> ()
                }
                frame 87 {
                }
                frame 88 {
                  n3311 = local write "S 90"(w4489) -> ()
                }
                frame 89 {
                  n3312 = local write "S 91"(w4490) -> ()
                }
                frame 90 {
                  n3313 = local write "S 92"(w4491) -> ()
                }
                frame 91 {
                  n3314 = local write "S 93"(w4492) -> ()
                }
                frame 92 {
                  n3315 = local write "S 94"(w4493) -> ()
                }
                frame 93 {
                  n3316 = local write "S 95"(w4494) -> ()
                }
                frame 94 {
                  n3317 = local write "S 96"(w4495) -> ()
                }
                frame 95 {
                  n3318 = local write "S 97"(w4496) -> ()
                }
                frame 96 {
                  n3319 = local write "S 98"(w4497) -> ()
                }
                frame 97 {
                  n3320 = local write "S 99"(w4498) -> ()
                }
                frame 98 {
                  n3321 = local write "S 100"(w4499) -> ()
                }
                frame 99 {
                  n3322 = local write "S 101"(w4500) -> ()
                }
                frame 100 {
                  n3323 = local write "S 102"(w4501) -> ()
                }
                frame 101 {
                  n3324 = local write "S 103"(w4502) -> ()
                }
                frame 102 {
                  n3325 = local write "S 104"(w4503) -> ()
                }
                frame 103 {
                  n3326 = local write "S 105"(w4504) -> ()
                }
                frame 104 {
                  n3327 = local write "S 106"(w4505) -> ()
                }
                frame 105 {
                }
                frame 106 {
                  n3328 = property on="OK Button 17" class="Bool (strict)"("Boolean Text.Text"=w4506) -> ()  [unwired: 2 in, 2 out]
                }
                frame 107 {
                  n3329 = property on="OK Button 16" class="Bool (strict)"("Boolean Text.Text"=w4507) -> ()  [unwired: 2 in, 2 out]
                }
                frame 108 {
                  n3330 = property on="TITTLE" class="Str"("Caption.Text"=w4508) -> ()  [unwired: 2 in, 2 out]
                }
                frame 109 {
                  "String 30" <- w4509
                }
                frame 110 {
                  n3331 = property on="Test Date" class="Str"("Caption.Text"=w4510) -> ()  [unwired: 2 in, 2 out]
                  "String 31" <- w4510
                }
                frame 111 {
                  n3332 = property on="Sample ID" class="Str"("Caption.Text"=w4511) -> ()  [unwired: 2 in, 2 out]
                  "String 32" <- w4511
                }
                frame 112 {
                  n3333 = property on="Tested by" class="Str"("Caption.Text"=w4512) -> ()  [unwired: 2 in, 2 out]
                  "String 33" <- w4512
                }
                frame 113 {
                  n3334 = property on="System Configured Printers 2" class="Arr (strict)"("Caption.Text"=w4513) -> ()  [unwired: 2 in, 2 out]
                }
                frame 114 {
                  n3335 = property on="Selected Printer" class="Str"("Caption.Text"=w4514) -> ()  [unwired: 2 in, 2 out]
                }
                frame 115 {
                  n3336 = property on="Select Printer 3" class="DigNum (strict)"("Caption.Text"=w4515) -> ()  [unwired: 2 in, 2 out]
                }
                frame 116 {
                  n3337 = property on="Print" class="Bool (strict)"("Boolean Text.Text"=w4516) -> ()  [unwired: 2 in, 2 out]
                }
                frame 117 {
                  "String 41" <- w4517
                }
                frame 118 {
                  n3338 = property on="tested by" class="Str"("Caption.Text"=w4518) -> ()  [unwired: 2 in, 2 out]
                }
                frame 119 {
                }
                frame 120 {
                  n3339 = property on="Export" class="Bool (strict)"("Boolean Text.Text"=w4519) -> ()  [unwired: 2 in, 2 out]
                }
                frame 121 {
                }
                frame 122 {
                }
                frame 123 {
                  n3340 = property on="Select File Type" class="Enum (strict)"("Caption.Text"=w4522) -> ()  [unwired: 2 in, 2 out]
                }
                frame 124 {
                  n3341 = property on="s.NO" class="Str"("Caption.Text"=w4523) -> ()  [unwired: 2 in, 2 out]
                  "String 45" <- w4523
                }
                frame 125 {
                  n3342 = property on="trip1 8" class="Bool (strict)"("Boolean Text.Text"=w4524) -> ()  [unwired: 2 in, 2 out]
                }
                frame 126, Default {
                }
              }
            }
          }
          frame #1 {
            w4532 = TRUE ("Visible")
            n3343 = local read "S 91"() -> (w4549:string)
            n3344 = local read "S 90"() -> (w4548:string)
            n3345 = local read "S 88"() -> (w4547:string)
            n3346 = property on="File Path" class="Path"("Caption.Text"=w4548) -> ()  [unwired: 2 in, 2 out]
            n3347 = local read "S 71"() -> (w4542:string)
            n3348 = local read "S 86"() -> (w4544:string)
            n3349 = local read "S 85"() -> (w4545:string)
            n3350 = local read "S 87"() -> (w4543:string)
            n3351 = local read "S 84"() -> (w4546:string)
            n3352 = local read "S 103"() -> (w4531:string)
            n3353 = local read "S 104"() -> (w4530:string)
            n3354 = property on="Password" class="Str"("Caption.Text"=w4545) -> ()  [unwired: 2 in, 2 out]
            n3355 = property on="EDIT" class="Bool (strict)"("Boolean Text.Text"=w4542) -> ()  [unwired: 2 in, 2 out]
            n3356 = property on="SAVE" class="Bool (strict)"("Boolean Text.Text"=w4546) -> ()  [unwired: 2 in, 2 out]
            n3357 = Build Array(w4531, w4530) -> (w4529:string[])
            n3358 = property on="Heater Button" class="Bool (strict)"("Strings [4]"=w4529) -> ()  [unwired: 2 in, 2 out]
            n3359 = local read "S 92"() -> (w4541:string)
            n3360 = local read "S 93"() -> (w4540:string)
            n3361 = local read "S 105"() -> (w4527:string)
            n3362 = local read "S 106"() -> (w4526:string)
            n3363 = Build Array(w4541, w4540) -> ()  [unwired: 1 out]
            n3364 = Build Array(w4527, w4526) -> (w4528:string[])
            n3365 = local read "S 95"() -> (w4538:string)
            n3366 = local read "S 94"() -> (w4539:string)
            n3367 = local read "bs"() -> (w4554:string)
            n3368 = local read "as"() -> (w4555:string)
            n3369 = property on="Humidity" class="Bool (strict)"("Strings [4]"=w4528) -> ()  [unwired: 2 in, 2 out]
            n3370 = Concatenate Strings(w4554, "\r", w4555) -> ()  [unwired: 1 out]
            n3371 = property on="Rh After" class="DigNum (strict)"("Caption.Size to Text?"=TRUE ("Caption.Size to Text")) -> ()  [unwired: 2 in, 2 out]
            n3372 = local read "S 48"() -> (w4578:string)
            n3373 = local read "S 50"() -> (w4576:string)
            n3374 = local read "S 51"() -> (w4575:string)
